vi "LAS-CTS_LaserEnergyReader.vi"() -> ()   [LabVIEW 2024]
uses:
  <vilib>/Analysis/baseanly.llb/Mean (DBL).vi
  <vilib>/Utility/file.llb/Write Delimited Spreadsheet (DBL).vi
  <vilib>/httpClient/LabVIEWHTTPClient.lvlib
  <vilib>/Analysis/NI_AALBase.lvlib
panel:
  out "Avg. Laser Energy (uJ)":dbl format="%.2f"
  out "Waveform Graph":dbl[](graph)
  in  "file path (dialog if empty)":path
  in  "Number of Pulses":i32
  out "number of measurements":i32
  out "Laser Energy (uJ)":dbl
  in  "VISA resource name":refnum<visa-resource-name>
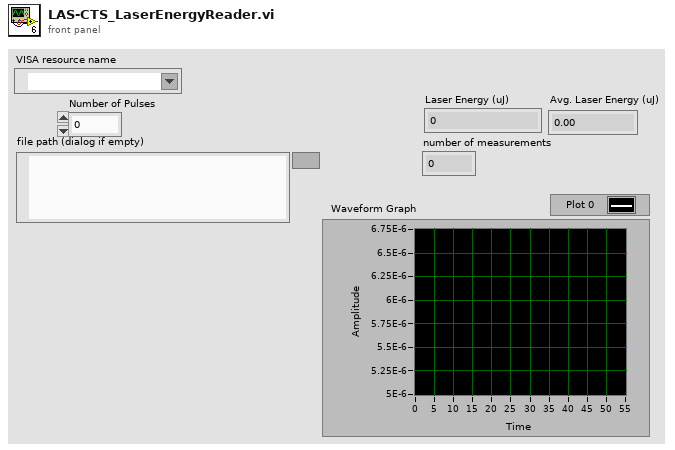
[diagram p1: front panel]
types:
  T1 = typedef "LabVIEWHTTPClient.lvlib/ClientHandle.ctl" = refnum<k1>
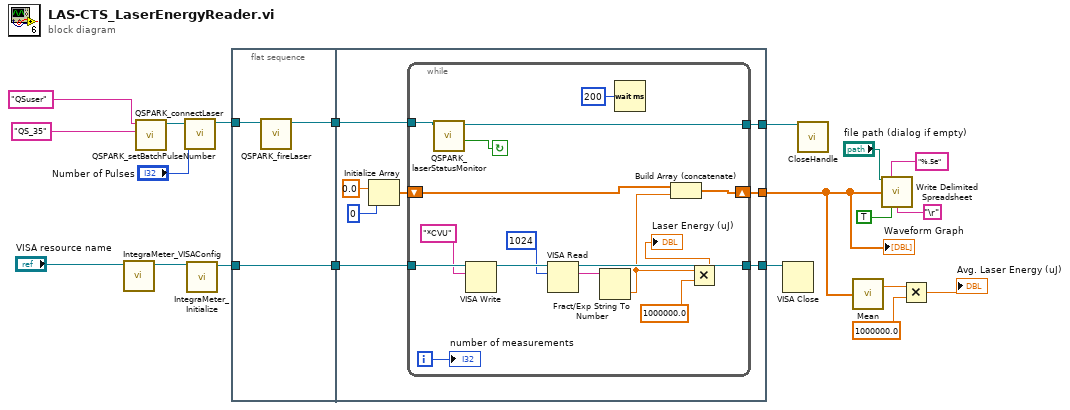
[diagram p0: block diagram]
diagram:
  n1 = call "IntegraMeter_VISAConfig.vi"("VISA resource name"="VISA resource name") -> ("reference out"=w20:refnum<visa-resource-name>)  [unwired: 9 in, 1 out]
  n2 = call "QSPARK_connectLaser.vi"("password"="QS_35", "username"="QSuser") -> ("client handle out"=w7:T1)  [unwired: 9 in]
  n3 = call "QSPARK_setBatchPulseNumber.vi"("Number of Pulses"="Number of Pulses", "client handle"=w7) -> ("client handle out"=w15:T1)  [unwired: 9 in]
  n4 = call "IntegraMeter_Initialize.vi"("VISA resource name"=w20) -> ("VISA resource name out"=w18:refnum<visa-resource-name>)  [unwired: 9 in, 1 out]
  n5 = flat-sequence {
    tunnel: w18 -> [w23]
    tunnel: [w23] -> w16
    tunnel: w15 -> [w22]
    tunnel: [w21] -> w13
    tunnel: [w30] -> w17
    tunnel: w16 -> [w31]
    tunnel: w13 -> [w29]
    tunnel: [w28] -> w12
    tunnel: [w24] -> w4
    frame #0 {
      n6 = call "QSPARK_fireLaser.vi"("client handle"=w22) -> ("client handle out"=w21:T1)  [unwired: 10 in]
    }
    frame #1 {
      n7 = Initialize Array(0.0 ("element"), 0 ("dimension size")) -> (w25:dbl[])
      n8 = while {
        tunnel: w31 -> [w47]
        tunnel: [w45] -> w30
        tunnel: w29 -> [w40]
        tunnel: [w39] -> w28
        shift-right: [w36] -> w24
        shift-left: w25 -> [w37]
        i -> [w41]
        stop <- w38 continue-if-true
        n9 = call "QSPARK_laserStatusMonitor.vi"("client handle"=w40) -> ("laser on?"=w38:bool, "client handle out"=w39:T1)  [unwired: 8 in, 1 out]
        n10 = VISA Write(VISA resource name=w47, write buffer="*CVU") -> (VISA resource name out=w46:refnum<visa-resource-name>)  [unwired: 1 in, 2 out]
        n11 = VISA Read(VISA resource name=w46, byte count=u32 1024) -> (VISA resource name out=w45:refnum<visa-resource-name>, read buffer=w42:string)  [unwired: 1 in, 2 out]
        n12 = Fract/Exp String To Number(string=w42) -> (number=w33:dbl)  [unwired: 3 in, 1 out]
        n13 = Wait (ms)(milliseconds to wait=u32 200 ("millisecond multiple")) -> ()  [unwired: 1 out]
        n14 = Build Array (concatenate)(w37, w33) -> (w36:dbl[])
        n15 = Multiply(x=w33, y=1000000.0) -> (x*y=→"Laser Energy (uJ)":dbl)
        "number of measurements" <- w41
      }
    }
  }
  n16 = VISA Close(VISA resource name=w17) -> ()  [unwired: 1 in, 1 out]
  n17 = call <vilib>:"CloseHandle.vi"("client handle"=w12) -> ()  [unwired: 14 in, 1 out]
  n18 = call-poly <vilib>:"Mean.vi"("X"=w4) -> ("mean"=w3:dbl)  [unwired: 1 out]
  n19 = call-poly <vilib>:"Write Delimited Spreadsheet.vi"("file path (dialog if empty)"="file path (dialog if empty)", "format (%.3f)"="%.5e", "1D data"=w4, "transpose? (no:F)"=TRUE, "delimiter (\\t)"="\r") -> ()  [unwired: 9 in, 2 out]
  n20 = Multiply(x=w3, y=1000000.0) -> (x*y=→"Avg. Laser Energy (uJ)":dbl)
  "Waveform Graph" <- w4
